vi "ReshapeTracksToDisplMatrix1.vi"(1 "Starting Pos":i32[](array[numeric]), 2 "# cols":i32, 3 "# rows":i32, 4 "Tracks (in columns)":dbl[][](array[numeric])) -> (0 "FR-TO-FR displ":dbl[][](array[numeric]))   [LabVIEW 2013]
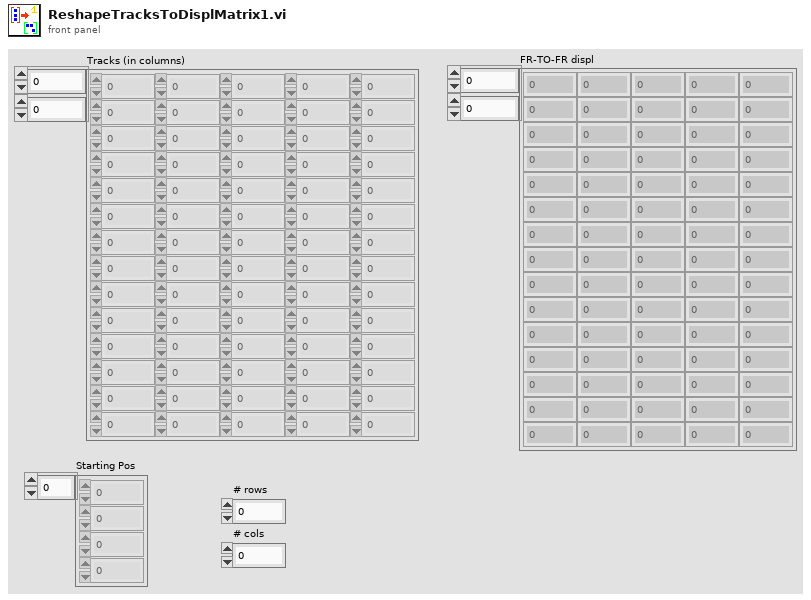
[diagram p1: front panel]
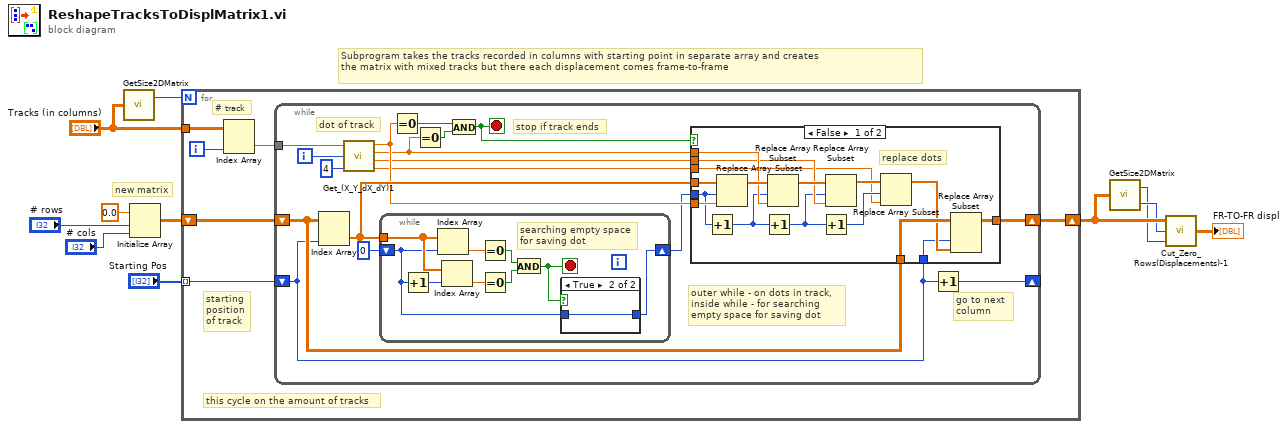
[diagram p0: block diagram]
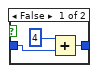
[diagram p3: hidden frame]
diagram:
  # "Subprogram takes the tracks recorded in columns with starting point in separate array and creates \nthe matrix with mixed tracks but there each displacement comes frame-to-frame"
  # "new matrix"
  n1 = call "GetSize2DMatrix.vi"("Array IN (2D)"="Tracks (in columns)") -> ("# Cols"=w8:i32)  [unwired: 1 out]
  n2 = Initialize Array(0.0 ("element"), "# rows", "# cols") -> (w6:dbl[][])
  n3 = for {
    N: w8 -> [_]
    tunnel: "Tracks (in columns)" -> [w17]
    shift-right: [w12] -> w4
    shift-left: w6 -> [w13]
    tunnel: "Starting Pos" -> [w14] mode=indexing
    i -> [w16]
    # "this cycle on the amount of tracks"
    # "starting \nposition\nof track"
    # "# track"
    n4 = Index Array(array=w17, index (col)=w16) -> (element=w15:dbl[])  [unwired: 1 in]
    n5 = while {
      tunnel: w15 -> [w34]
      shift-right: [w21] -> w12
      shift-left: w13 -> [w22]
      shift-right: [w19] -> _
      shift-left: w14 -> [w20]
      i -> [w33]
      stop <- w18 stop-if-true
      # "outer while - on dots in track,\ninside while - for searching \nempty space for saving dot"
      # "go to next \ncolumn"
      # "stop if track ends"
      # "dot of track"
      n6 = Index Array(array=w22, index (col)=w20) -> (element=w28:dbl[])  [unwired: 1 in]
      n7 = call "Get_(X_Y_dX_dY)1.vi"("(X,Y,dX,dY)"=w34, "index"=w33, "multiplier"=4 ("multiplayer")) -> ("X"=w27:dbl, "Y"=w25:dbl, "dX"=w24:dbl, "dY"=w23:dbl)
      n8 = while {
        tunnel: w28 -> [w58]
        shift-right: [w52] -> w26
        shift-left: 0 -> [w53]
        stop <- w54 stop-if-true
        # "searching empty space\nfor saving dot"
        n9 = Increment(x=w53) -> (x+1=w59:i32)
        n10 = Index Array(array=w58, index=w53) -> (element=w60:dbl)
        n11 = Index Array(array=w58, index=w59) -> (element=w57:dbl)
        n12 = Equal To 0?(x=w60) -> (x = 0?=w56:bool)
        n13 = Equal To 0?(x=w57) -> (x = 0?=w55:bool)
        n14 = And(x=w56, y=w55) -> (x .and. y?=w54:bool)
        n15 = case shown="True" w54 {
          tunnel: w53 -> [w62 w64]
          tunnel: [w63 w64] -> w52
          frame False {
            n16 = Add(x=4, y=w62) -> (x+y=w63:i32)
          }
          frame True {
          }
        }
      }
      n17 = Equal To 0?(x=w27) -> (x = 0?=w31:bool)
      n18 = Equal To 0?(x=w25) -> (x = 0?=w30:bool)
      n19 = And(x=w31, y=w30) -> (x .and. y?=w18:bool)
      n20 = case shown="False" w18 {
        tunnel: w28 -> [w50 _]
        tunnel: w27 -> [w49 _]
        tunnel: w26 -> [w47 _]
        tunnel: w25 -> [w46 _]
        tunnel: w24 -> [w43 _]
        tunnel: w23 -> [w39 _]
        tunnel: w22 -> [w38 w51]
        tunnel: [w36 w51] -> w21
        tunnel: w20 -> [w35 _]
        frame False {
          # "replace dots"
          n21 = Increment(x=w47) -> (x+1=w44:i32)
          n22 = Replace Array Subset(array=w50, new element=w49, index=w47) -> (w48:dbl[])
          n23 = Increment(x=w44) -> (x+1=w41:i32)
          n24 = Replace Array Subset(array=w48, new element=w46, index=w44) -> (w45:dbl[])
          n25 = Increment(x=w41) -> (x+1=w40:i32)
          n26 = Replace Array Subset(array=w45, new element=w43, index=w41) -> (w42:dbl[])
          n27 = Replace Array Subset(array=w42, new element=w39, index=w40) -> (w37:dbl[])
          n28 = Replace Array Subset(array=w38, new element=w37, index (col)=w35) -> (w36:dbl[][])  [unwired: 1 in]
        }
        frame True {
        }
      }
      n29 = Increment(x=w20) -> (x+1=w19:i32)
    }
  }
  n30 = call "GetSize2DMatrix.vi"("Array IN (2D)"=w4) -> ("# Cols"=w2:i32, "# Rows"=w3:i32)
  n31 = call "Cut_Zero_Rows(Displacements)-1.vi"("# Cols"=w2, "# Rows"=w3, "Array IN"=w4) -> ("Array OUT"=→"FR-TO-FR displ":dbl[][])
